vi "Kalman Calculation for balls.vi"(4 "R":T1=[[0.1, 0.0, 0.0], [0.0, 0.1, 0.0], [0.0, 0.0, 0.1]], 6 "intervalo":dbl=1.0, 8 "Pk-1|k-1":T1, 9 "x_k-1|k-1":T1=[[0.0, 0.0, 0.0], [0.0, 0.0, 0.0], [0.0, 0.0, 0.0]], 10 "z_k":T1, 11 "Use Observation":bool=TRUE) -> (1 "Conf":dbl, 2 "Pk|k":T1, 3 "x_k|k":T1)   [LabVIEW 2023]
uses:
  <vilib>/Analysis/Matrix/Datatypes/RealMatrix.ctl
  <vilib>/Analysis/_algsub.llb/Real Matrix Norm.vi
  <vilib>/Analysis/Matrix/Numeric/Multiply/Multiply - RM,RM.vi
  <vilib>/Analysis/Matrix/Numeric/Add/Add - RM,RM.vi
  <vilib>/Analysis/baseanly.llb/Real Inverse Matrix.vi
  <vilib>/Analysis/Matrix/Numeric/Subtract/Subtract - RM,RM.vi
  <vilib>/Analysis/Matrix/NI_Matrix.lvlib
  <vilib>/Analysis/NI_AALBase.lvlib
  <vilib>/Analysis/NI_AALPro.lvlib
panel:
  out "Inverse Matrix":T1
  out "K_k":T1
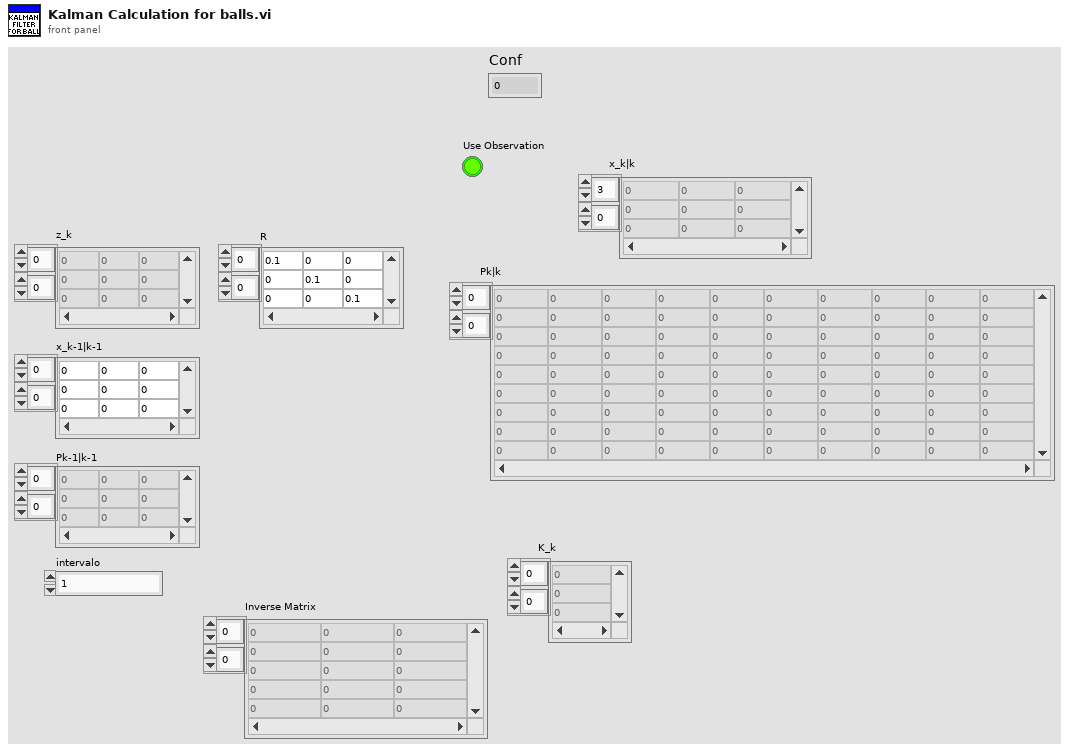
[diagram p1: front panel]
types:
  T1 = typedef "NI_Matrix.lvlib/RealMatrix.ctl" = dbl[][]
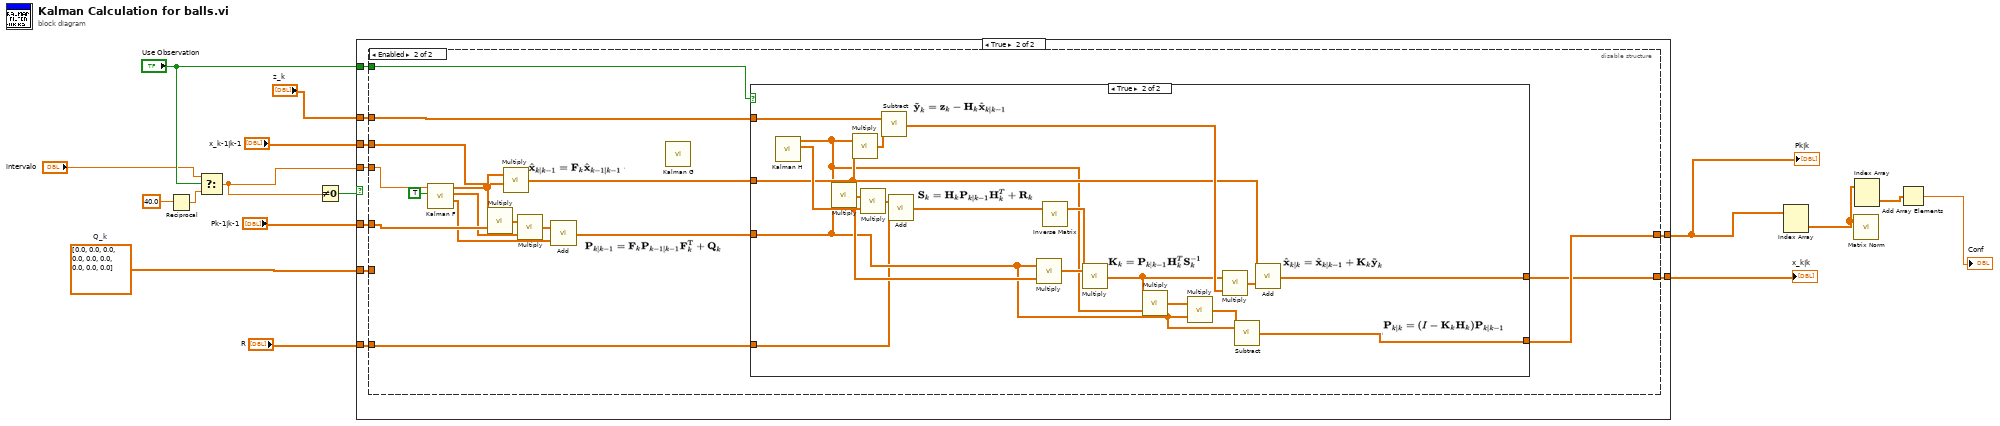
[diagram p0: block diagram]
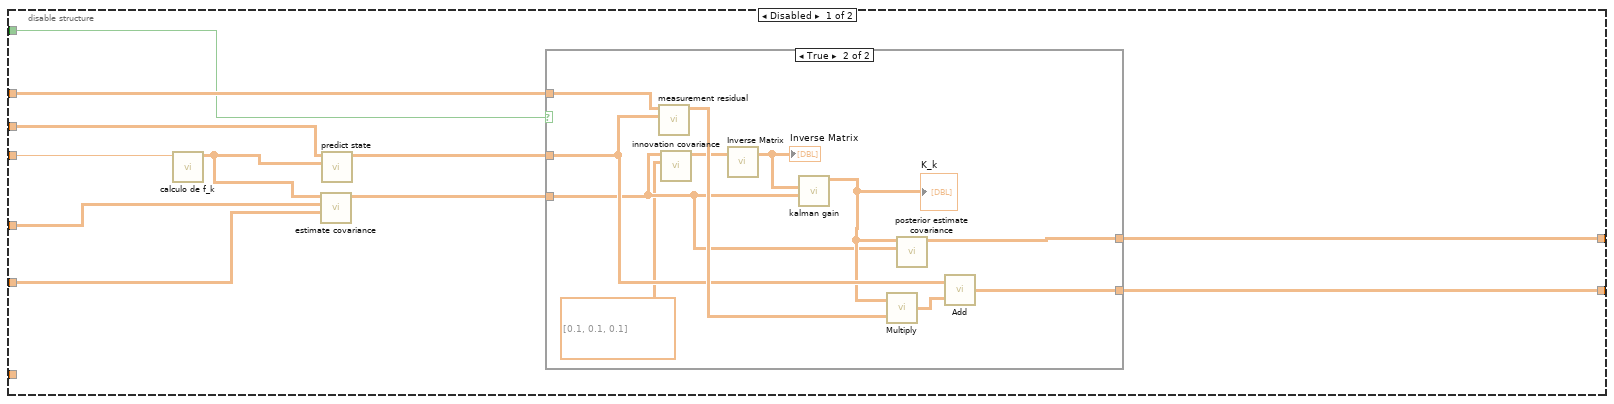
[diagram p3: hidden frame]
diagram:
  w12 = T1 [[0.0, 0.0, 0.0], [0.0, 0.0, 0.0], [0.0, 0.0, 0.0]]  # Q_k
  n1 = Reciprocal(x=40.0) -> (1/x=w2:dbl)
  n2 = Select(t="intervalo", s="Use Observation", f=w2) -> (s? t:f=w1:dbl)
  n3 = Not Equal To 0?(x=w1) -> (x != 0?=w13:bool)
  n4 = case shown="True" w13 {
    tunnel: w1 -> [_ w27]
    tunnel: [w18 w26] -> w6
    tunnel: "Pk-1|k-1" -> [w17 w25]
    tunnel: "x_k-1|k-1" -> [w18 w23]
    tunnel: [w17 w24] -> w14
    tunnel: w12 -> [_ w22]
    tunnel: "z_k" -> [_ w21]
    tunnel: "Use Observation" -> [_ w20]
    tunnel: "R" -> [_ w19]
    frame False {
    }
    frame True {
      n5 = disable-structure shown="Enabled" {
        disable-tunnel: w27 -> [w38 w67]
        disable-tunnel: [w35 w58] -> w26
        disable-tunnel: w25 -> [w34 w66]
        disable-tunnel: [w33 w59] -> w24
        disable-tunnel: w23 -> [w32 w56]
        disable-tunnel: w22 -> [w30 _]
        disable-tunnel: w21 -> [w29 w53]
        disable-tunnel: w20 -> [w28 w54]
        disable-tunnel: w19 -> [_ w55]
        frame Disabled {
          n6 = call "calculo de f_k.vi"("iteração"=w38) -> ("F_k"=w31:T1)  [unwired: 10 in]
          n7 = call "estimate covariance.vi"("Q_k"=w30, "Pk-1|k-1"=w34, "F_k"=w31) -> ("Pk|k-1"=w36:T1)  [unwired: 8 in]
          n8 = call "predict state.vi"("F_k"=w31, "x_k-1|k-1"=w32) -> ("x_k|k-1"=w37:T1)  [unwired: 9 in]
          n9 = case shown="True" w28 {
            tunnel: [w40 w50] -> w35
            tunnel: w37 -> [w40 w48]
            tunnel: [w39 w45] -> w33
            tunnel: w36 -> [w39 w43]
            tunnel: w29 -> [_ w42]
            frame False {
            }
            frame True {
              n10 = call "measurement residual.vi"("x_k|k-1"=w48, "z_k"=w42) -> ("y~_k"=w49:T1)  [unwired: 9 in]
              n11 = call "innovation covariance.vi"("R"=T1 [[0.1, 0.1, 0.1]], "Pk|k-1"=w43) -> ("S_k"=w47:T1)  [unwired: 8 in, 1 out]
              n12 = call-poly <vilib>:"Inverse Matrix.vi"("Input Matrix"=w47) -> ("Inverse Matrix"=w46:T1)  [unwired: 1 in, 1 out]
              "Inverse Matrix" <- w46
              n13 = call "kalman gain.vi"("Pk|k-1"=w43, "S^-1"=w46) -> ("K_k"=w44:T1)  [unwired: 9 in]
              "K_k" <- w44
              n14 = call-poly <vilib>:"Multiply.vi"("Real Matrix B"=w49, "Real Matrix A"=w44) -> ("A * B"=w51:T1)
              n15 = call "posterior estimate covariance.vi"("Pk|k-1"=w43, "K_k"=w44) -> ("Pk|k"=w45:T1)  [unwired: 9 in]
              n16 = call-poly <vilib>:"Add.vi"("Real Matrix B"=w51, "Real Matrix A"=w48) -> ("A + B"=w50:T1)
            }
          }
        }
        frame Enabled {
          n17 = call "Kalman F.vi"("Ball?"=TRUE, "intervalo"=w67) -> ("Q"=w62:T1, "F'"=w64:T1, "F"=w57:T1)  [unwired: 7 in]
          n18 = call-poly <vilib>:"Multiply.vi"("Real Matrix B"=w66, "Real Matrix A"=w57) -> ("A * B"=w65:T1)
          n19 = call-poly <vilib>:"Multiply.vi"("Real Matrix B"=w56, "Real Matrix A"=w57) -> ("A * B"=w61:T1)
          n20 = call-poly <vilib>:"Multiply.vi"("Real Matrix B"=w64, "Real Matrix A"=w65) -> ("A * B"=w63:T1)
          n21 = call-poly <vilib>:"Add.vi"("Real Matrix B"=w62, "Real Matrix A"=w63) -> ("A + B"=w60:T1)
          n22 = call "Kalman G.vi"() -> ()  [unwired: 11 in, 1 out]
          n23 = case shown="True" w54 {
            tunnel: w53 -> [_ w88]
            tunnel: w61 -> [w69 w78]
            tunnel: w60 -> [w68 w74]
            tunnel: [w68 w72] -> w59
            tunnel: [w69 w71] -> w58
            tunnel: w55 -> [_ w70]
            frame False {
            }
            frame True {
              n24 = call "Kalman H.vi"() -> ("H'"=w83:T1, "H"=w76:T1)  [unwired: 10 in]
              n25 = call-poly <vilib>:"Multiply.vi"("Real Matrix B"=w74, "Real Matrix A"=w76) -> ("A * B"=w86:T1)
              n26 = call-poly <vilib>:"Multiply.vi"("Real Matrix B"=w78, "Real Matrix A"=w76) -> ("A * B"=w87:T1)
              n27 = call-poly <vilib>:"Multiply.vi"("Real Matrix B"=w83, "Real Matrix A"=w86) -> ("A * B"=w85:T1)
              n28 = call-poly <vilib>:"Subtract.vi"("Real Matrix B"=w87, "Real Matrix A"=w88) -> ("A - B"=w80:T1)
              n29 = call-poly <vilib>:"Add.vi"("Real Matrix B"=w70, "Real Matrix A"=w85) -> ("A + B"=w84:T1)
              n30 = call-poly <vilib>:"Multiply.vi"("Real Matrix B"=w83, "Real Matrix A"=w74) -> ("A * B"=w82:T1)
              n31 = call-poly <vilib>:"Inverse Matrix.vi"("Input Matrix"=w84) -> ("Inverse Matrix"=w81:T1)  [unwired: 1 in, 1 out]
              n32 = call-poly <vilib>:"Multiply.vi"("Real Matrix B"=w81, "Real Matrix A"=w82) -> ("A * B"=w77:T1)
              n33 = call-poly <vilib>:"Multiply.vi"("Real Matrix B"=w76, "Real Matrix A"=w77) -> ("A * B"=w75:T1)
              n34 = call-poly <vilib>:"Multiply.vi"("Real Matrix B"=w74, "Real Matrix A"=w75) -> ("A * B"=w73:T1)
              n35 = call-poly <vilib>:"Multiply.vi"("Real Matrix B"=w80, "Real Matrix A"=w77) -> ("A * B"=w79:T1)
              n36 = call-poly <vilib>:"Subtract.vi"("Real Matrix B"=w73, "Real Matrix A"=w74) -> ("A - B"=w72:T1)
              n37 = call-poly <vilib>:"Add.vi"("Real Matrix B"=w79, "Real Matrix A"=w78) -> ("A + B"=w71:T1)
            }
          }
        }
      }
    }
  }
  "Pk|k" <- w14
  "x_k|k" <- w6
  n38 = Index Array(array=w14) -> (element=w9:T1)  [unwired: 2 in]
  n39 = call-poly <vilib>:"Matrix Norm.vi"("Input Matrix"=w9) -> ()  [unwired: 1 in, 2 out]
  n40 = Index Array(array=w9) -> (element=w8:T1)  [unwired: 2 in]
  n41 = Add Array Elements(numeric array=w8) -> (sum=→"Conf":dbl)
